vi "write_lockin_FP_DSC.vi"(8 "error in (no error)":errorcluster, 11 "front panel":T1 {"Channels: AO"."AO f (Hz)" min=0.001 max=10000.0; "Channels: AO"."AO DC (V)" format="%#_6p"; "Channels: AO"."AO amp (V)" format="%#_6p"; "Channels: Lockin"."REF phi (deg)" format="%#_3g"}) -> (0 "error out":errorcluster)   [LabVIEW 2016]
uses:
  Typedefs/Front Panel Cluster.ctl
  Typedefs/AO.config-array.ctl
  Typedefs/AO.config-cluster.ctl
  Typedefs/446xAO-enum.ctl
  Typedefs/AI.config-array.ctl
  Typedefs/AI.config-cluster.ctl
  Typedefs/AI.coupling-enum.ctl
  Typedefs/446xAI-enum.ctl
  Typedefs/AO-cluster.ctl
  Typedefs/AO_Amp-array.ctl
  Typedefs/AO_DC-array.ctl
  Typedefs/AO_f-array.ctl
  Typedefs/AO_phi-array.ctl
  Typedefs/Function-array.ctl
  Typedefs/Function-enum.ctl
  Typedefs/REF-cluster.ctl
  Typedefs/REF_f-array.ctl
  Typedefs/REF_phi-array.ctl
  Typedefs/DAQType-enum.ctl
  Typedefs/AmplifierType-enum.ctl
  <vilib>/addons/_JKI.lib/Serialization/JSON/JKI JSON Serialization.lvlib
panel:
  # "0"
  # "1"
  # "2"
  # "3"
  # "4"
  # "5"
  # "6"
  # "7"
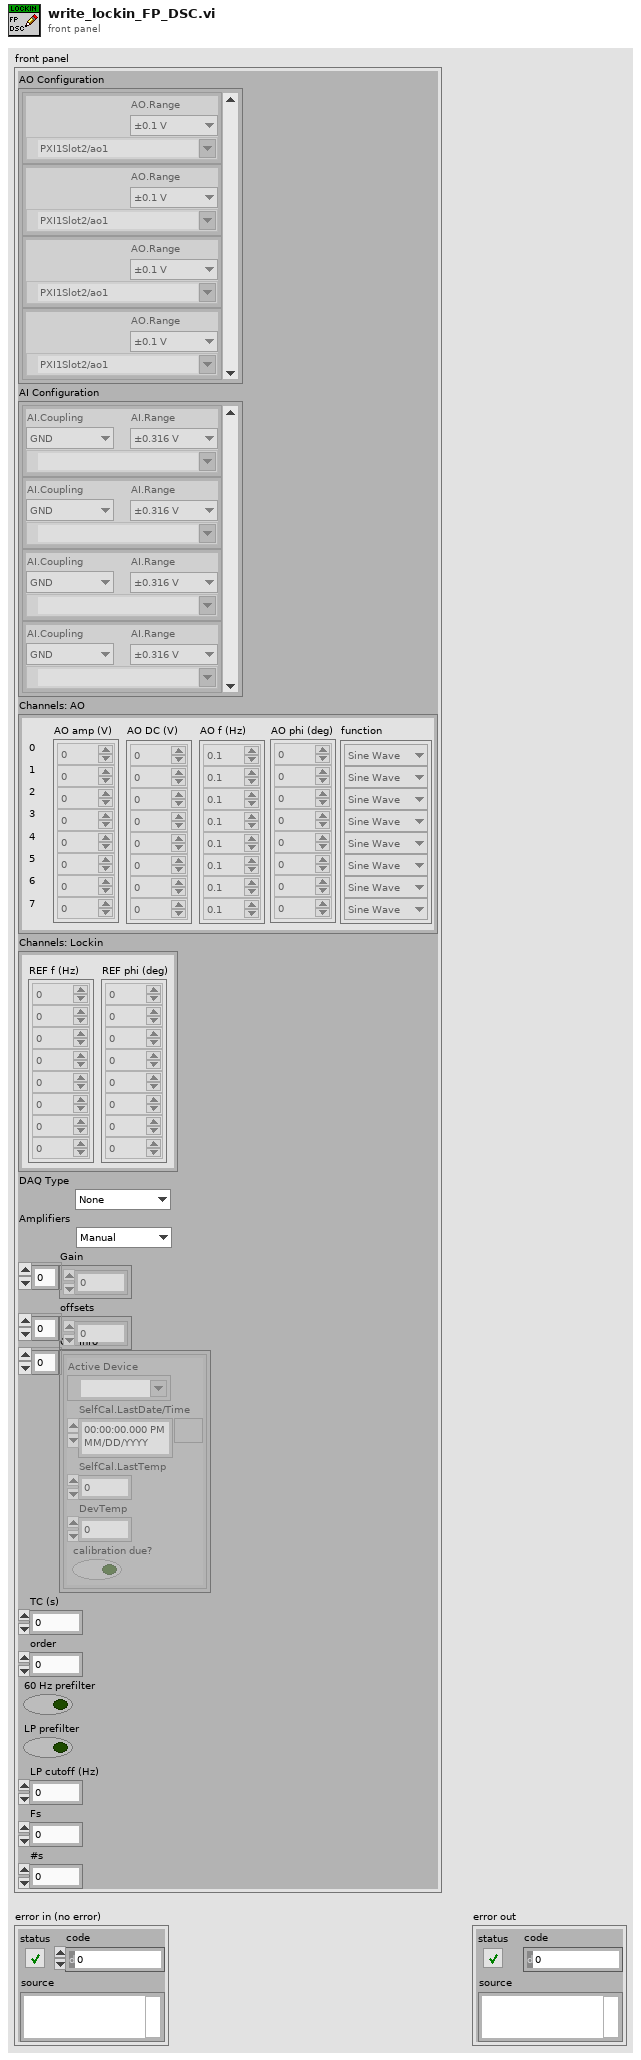
[diagram p1: front panel]
types:
  T1 = typedef "Front Panel Cluster.ctl" = cluster{"AO Configuration":T2, "AI Configuration":T5, "Channels: AO":T9, "Channels: Lockin":T16, "DAQ Type":T19, "Amplifiers":T20, "Gain":dbl[], "offsets":dbl[], "Cal Info":cluster{"Active Device":tag, "SelfCal.LastDate/Time":timestamp, "SelfCal.LastTemp":dbl, "DevTemp":dbl, "calibration due?":bool}[], "TC (s)":dbl, "order":i32, "60 Hz prefilter":bool, "LP prefilter":bool, "LP cutoff (Hz)":dbl, "Fs":i32, "#s":i32}
  T2 = typedef "AO.config-array.ctl" = T3[]
  T3 = typedef "AO.config-cluster.ctl" = cluster{"AO.Range":T4, "AO.channels":tag}
  T4 = typedef "446xAO-enum.ctl" = enum16{"±0.1 V", "±1.0 V", "±10.0 V"}
  T5 = typedef "AI.config-array.ctl" = T6[]
  T6 = typedef "AI.config-cluster.ctl" = cluster{"AI.Coupling":T7, "AI.channels":tag, "AI.Range":T8}
  T7 = typedef "AI.coupling-enum.ctl" = enum16{"AC", "DC", "GND"}
  T8 = typedef "446xAI-enum.ctl" = enum16{"±0.316 V", "±1.00 V", "±3.16 V", "±10.0 V", "±31.6 V", "±42.4 V"}
  T9 = typedef "AO-cluster.ctl" = cluster{"AO amp (V)":T10, "AO DC (V)":T11, "AO f (Hz)":T12, "AO phi (deg)":T13, "function":T14}
  T10 = typedef "AO_Amp-array.ctl" = dbl[]
  T11 = typedef "AO_DC-array.ctl" = dbl[]
  T12 = typedef "AO_f-array.ctl" = dbl[]
  T13 = typedef "AO_phi-array.ctl" = dbl[]
  T14 = typedef "Function-array.ctl" = T15[]
  T15 = typedef "Function-enum.ctl" = enum16{"Sine Wave", "Triangle Wave", "Square Wave", "Sawtooth Wave"}
  T16 = typedef "REF-cluster.ctl" = cluster{"REF f (Hz)":T17, "REF phi (deg)":T18}
  T17 = typedef "REF_f-array.ctl" = dbl[]
  T18 = typedef "REF_phi-array.ctl" = dbl[]
  T19 = typedef "DAQType-enum.ctl" = enum16{"None", "USB 4431", "PXI 446x"}
  T20 = typedef "AmplifierType-enum.ctl" = enum16{"Manual", "Krohn Hite", "Femto"}
  T21 = cluster{"AO Configuration":cluster{"AO.Range":T4, "AO.channels":string}[], "AI Configuration":cluster{"AI.Coupling":T7, "AI.channels":string, "AI.Range":T8}[], "Channels: AO":T9, "Channels: Lockin":T16, "DAQ Type":T19, "Amplifiers":T20, "Gain":dbl[], "offsets":dbl[], "Cal Info":cluster{"Active Device":string, "SelfCal.LastDate/Time":timestamp, "SelfCal.LastTemp":dbl, "DevTemp":dbl, "calibration due?":bool}[], "TC (s)":dbl, "order":i32, "60 Hz prefilter":bool, "LP prefilter":bool, "LP cutoff (Hz)":dbl, "Fs":i32, "#s":i32}
  T22 = cluster{"Active Device":tag, "SelfCal.LastDate/Time":timestamp, "SelfCal.LastTemp":dbl, "DevTemp":dbl, "calibration due?":bool}[]
  T23 = cluster{"AI.Coupling":T7, "AI.channels":string, "AI.Range":T8}
  T24 = cluster{"Active Device":string, "SelfCal.LastDate/Time":timestamp, "SelfCal.LastTemp":dbl, "DevTemp":dbl, "calibration due?":bool}
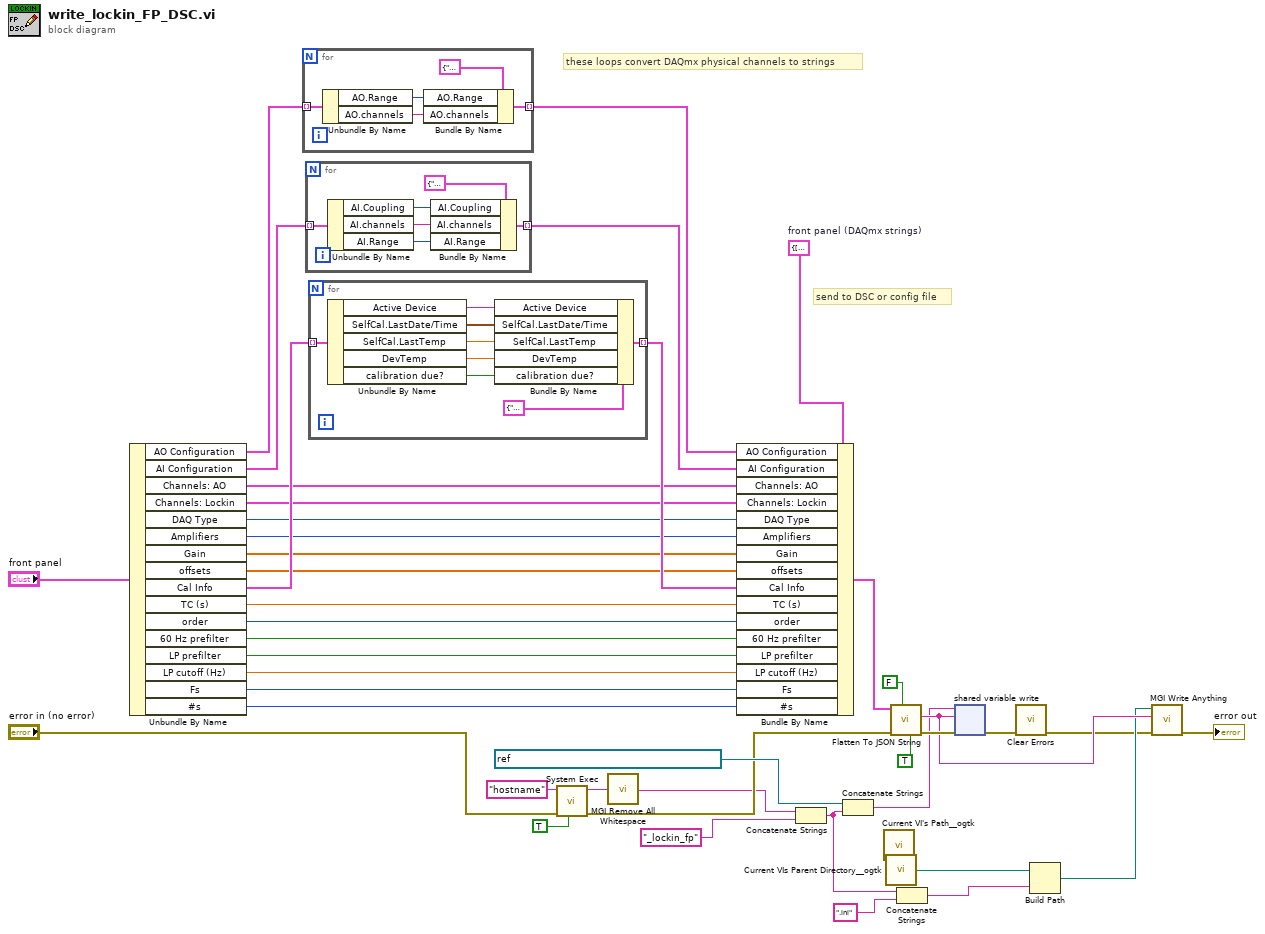
[diagram p0: block diagram]
diagram:
  w20 = T21 {"AO Configuration"=[], "AI Configuration"=[], "Channels: AO"={"AO amp (V)"=[], "AO DC (V)"=[], "AO f (Hz)"=[], "AO phi (deg)"=[], "function"=[]}, "Channels: Lockin"={"REF f (Hz)"=[], "REF phi (deg)"=[]}, "DAQ Type"=enum."None", "Amplifiers"=enum."Manual", "Gain"=[], "offsets"=[], "Cal Info"=[], "TC (s)"=0.0, "order"=0, "60 Hz prefilter"=FALSE, "LP prefilter"=FALSE, "LP cutoff (Hz)"=0.0, "Fs"=0, "#s"=0}  # front panel (DAQmx strings)
  # "these loops convert DAQmx physical channels to strings"
  # "send to DSC or config file"
  n1 = Unbundle By Name("front panel") -> ("AO Configuration"=w21:T2, "AI Configuration"=w22:T5, "Channels: AO"=w23:T9, "Channels: Lockin"=w24:T16, "DAQ Type"=w25:T19, "Amplifiers"=w26:T20, "Gain"=w27:dbl[], "offsets"=w28:dbl[], "Cal Info"=w29:T22, "TC (s)"=w30:dbl, "order"=w31:i32, "60 Hz prefilter"=w32:bool, "LP prefilter"=w33:bool, "LP cutoff (Hz)"=w34:dbl, "Fs"=w35:i32, "#s"=w36:i32)
  n2 = for {
    tunnel: w21 -> [w48] mode=indexing
    tunnel: [w46] -> w39 mode=indexing
    n3 = Unbundle By Name(w48) -> ("AO.Range"=w47:T4, "AO.channels"=w44:tag)
    n4 = Bundle By Name(cluster=cluster{"AO.Range":T4, "AO.channels":string} {"AO.Range"=enum."±0.1 V", "AO.channels"=""}, "AO.Range"=w47, "AO.channels"=w44) -> (w46:cluster{"AO.Range":T4, "AO.channels":string})
  }
  n5 = for {
    tunnel: w22 -> [w54] mode=indexing
    tunnel: [w53] -> w38 mode=indexing
    n6 = Unbundle By Name(w54) -> ("AI.Coupling"=w49:T7, "AI.channels"=w50:tag, "AI.Range"=w51:T8)
    n7 = Bundle By Name(cluster=T23 {"AI.Coupling"=enum."AC", "AI.channels"="", "AI.Range"=enum."±0.316 V"}, "AI.Coupling"=w49, "AI.channels"=w50, "AI.Range"=w51) -> (w53:T23)
  }
  n8 = for {
    tunnel: w29 -> [w61] mode=indexing
    tunnel: [w62] -> w37 mode=indexing
    n9 = Unbundle By Name(w61) -> ("Active Device"=w55:tag, "SelfCal.LastDate/Time"=w56:timestamp, "SelfCal.LastTemp"=w57:dbl, "DevTemp"=w58:dbl, "calibration due?"=w59:bool)
    n10 = Bundle By Name(cluster=T24 {"Active Device"="", "SelfCal.LastDate/Time"=timestamp(0 s since 1904-01-01), "SelfCal.LastTemp"=0.0, "DevTemp"=0.0, "calibration due?"=FALSE}, "Active Device"=w55, "SelfCal.LastDate/Time"=w56, "SelfCal.LastTemp"=w57, "DevTemp"=w58, "calibration due?"=w59) -> (w62:T24)
  }
  n11 = call <vilib>:"System Exec.vi"("run minimized? (F)"=TRUE, "error in (no error)"="error in (no error)", "command line"="hostname") -> ("error out"=w3:errorcluster, "standard output"=w4:string)  [unwired: 5 in, 2 out]
  n12 = call <userlib>:"MGI Remove All Whitespace.vi"("String"=w4) -> ("Trimmed String"=w2:string)
  n13 = Bundle By Name(cluster=w20, "AO Configuration"=w39, "AI Configuration"=w38, "Channels: AO"=w23, "Channels: Lockin"=w24, "DAQ Type"=w25, "Amplifiers"=w26, "Gain"=w27, "offsets"=w28, "Cal Info"=w37, "TC (s)"=w30, "order"=w31, "60 Hz prefilter"=w32, "LP prefilter"=w33, "LP cutoff (Hz)"=w34, "Fs"=w35, "#s"=w36) -> (w18:T21)
  n14 = Concatenate Strings(w2, "_lockin_fp" ("regular expression")) -> (w9:string)
  n15 = Concatenate Strings(refnum<k21> "ni.var.psp://housesoftheholy/lockins/" ("shared variable refnum in"), w9) -> (w11:string)
  n16 = call <userlib>:"Current VI's Path__ogtk.vi"() -> ()  [unwired: 1 in, 1 out]
  n17 = call <userlib>:"Current VIs Parent Directory__ogtk.vi"() -> ("Parent Directory (+ Relative)"=w17:path)  [unwired: 5 in]
  n18 = call <vilib>:"Flatten To JSON String.vi"("Enums As String (F)"=TRUE, "Multiline (T)"=FALSE, "error in (no error)"=w3, "Variant"=w18) -> ("error out"=w42:errorcluster, "JSON String"=w16:string)  [unwired: 6 in]
  n19 = Concatenate Strings(w9, ".ini" ("name or relative path")) -> (w8:string)
  n20 = shared-variable-write(w11, w42, w16) -> (w15:errorcluster)  [unwired: 1 out]
  n21 = call <vilib>:"Clear Errors.vi"("error in (no error)"=w15) -> ("error out"=w1:errorcluster)  [unwired: 5 in, 1 out]
  n22 = Build Path(base path=w17, name or relative path=w8) -> (appended path=w13:path)
  n23 = call <userlib>:"MGI Write Anything.vi"("Error In"=w1, "Anything"=w16, "Path (dialog)"=w13) -> ("Error Out"=→"error out":errorcluster)  [unwired: 6 in, 2 out]
